vi "OpenMasterWebPages.vi"   [LabVIEW 2015]
uses:
  vi.lib/Platform/browser.llb/Open URL in Default Browser (string).vi
  _ROSDefinition.vi
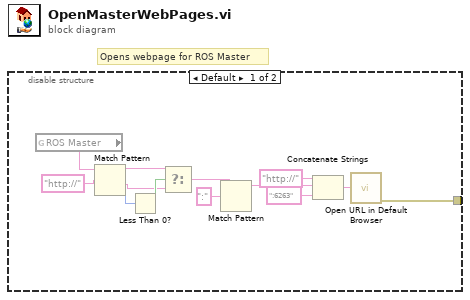
[diagram p0: block diagram]
diagram:
  # "Opens webpage for ROS Master"
  n1 = disable-structure shown="Default" {
    disable-tunnel: [w6 _] -> _
    frame condition #0 {
      n2 = global read "_ROSDefinition.vi" "ROS Master"() -> (w7:string)
      n3 = Match Pattern(string=w7, regular expression="http://" ("string")) -> (before substring=w3:string, after substring=w2:string, offset past match=w5:i32)  [unwired: 1 in, 1 out]
      n4 = Less Than 0?(x=w5) -> (x < 0?=w4:bool)
      n5 = Select(t=w3, s=w4, f=w2) -> (s? t:f=w1:string)
      n6 = Match Pattern(string=w1, regular expression=":") -> (before substring=w12:string)  [unwired: 1 in, 3 out]
      n7 = Concatenate Strings("http://" ("string"), w12, ":6263" ("string")) -> (w10:string)
      n8 = call-poly "Open URL in Default Browser.vi"("URL"=w10) -> ("error out"=w6:errorcluster)  [unwired: 5 in, 1 out]
    }
    frame condition #1 (active) {
    }
  }
